vi "Task Done.vi"(8 "error in (no error)":errorcluster, 11 "NI PWM Output in":refnum<class "NI PWM Output.lvclass">) -> (0 "error out":errorcluster, 3 "NI PWM Output out":refnum<class "NI PWM Output.lvclass">)   [LabVIEW 2023, in "HardwareAbstractionLayer_LVOOP.lvlib" / "NI PWM Output.lvclass"]
uses:
  NI PWM Output.lvclass
  NI PWM Output.lvclass/NI PWM Output.ctl
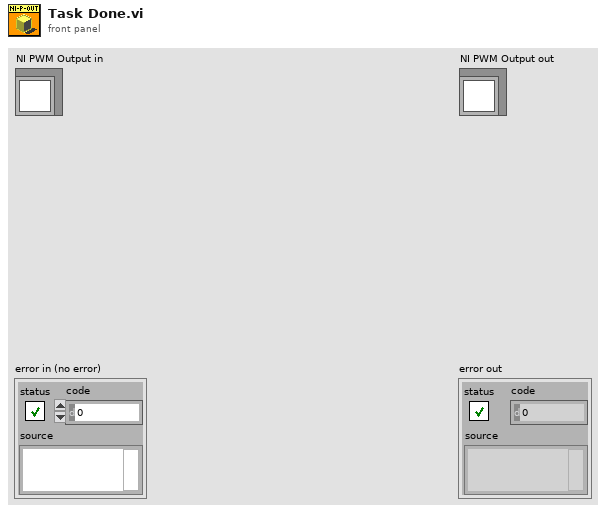
[diagram p1: front panel]
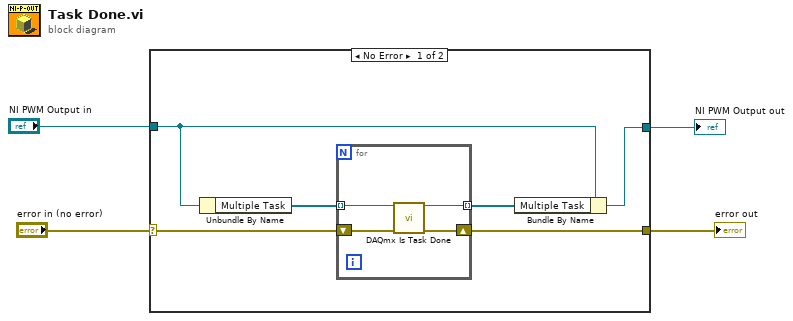
[diagram p0: block diagram]
diagram:
  n1 = case shown="No Error" "error in (no error)" {
    selector: "error in (no error)" -> [w10 w15]
    tunnel: [w9 w15] -> w3
    tunnel: "NI PWM Output in" -> [w7 w16]
    tunnel: [w5 w16] -> w1
    frame No Error {
      n2 = Unbundle By Name(w7) -> ("Multiple Task"=w8:refnum<k21>[])
      n3 = for {
        shift-right: [w13] -> w9
        shift-left: w10 -> [w14]
        tunnel: w8 -> [w12] mode=indexing
        tunnel: [w11] -> w6 mode=indexing
        n4 = call <vilib>:"DAQmx Is Task Done.vi"("task/channels in"=w12, "error in"=w14) -> ("task out"=w11:refnum<k21>, "error out"=w13:errorcluster)  [unwired: 11 in, 1 out]
      }
      n5 = Bundle By Name(cluster=w7, "Multiple Task"=w6) -> (w5:refnum<class "NI PWM Output.lvclass">)
    }
    frame Error {
    }
  }
  "error out" <- w3
  "NI PWM Output out" <- w1
